vi "calculate_histogram.vi"(8 "error in (no error)":errorcluster, 9 "# bins [100]":i32=100, 10 "# std deviations for histogram width [1]":dbl=1.0, 11 "2D arr Intensity Graph":dbl[][](array[numeric])=array402x480[192960 elements]) -> (0 "error out":errorcluster, 1 "standard deviation":dbl format="%0.2f", 2 "mean":dbl format="%0.2f", 3 "Histogram Graph":T1(graph))   [LabVIEW 2019, in "graph_utilities.lvclass"]
uses:
  graph_utilities.lvclass
  <vilib>/Analysis/NI_AALPro.lvlib
  <vilib>/Analysis/NI_AALBase.lvlib
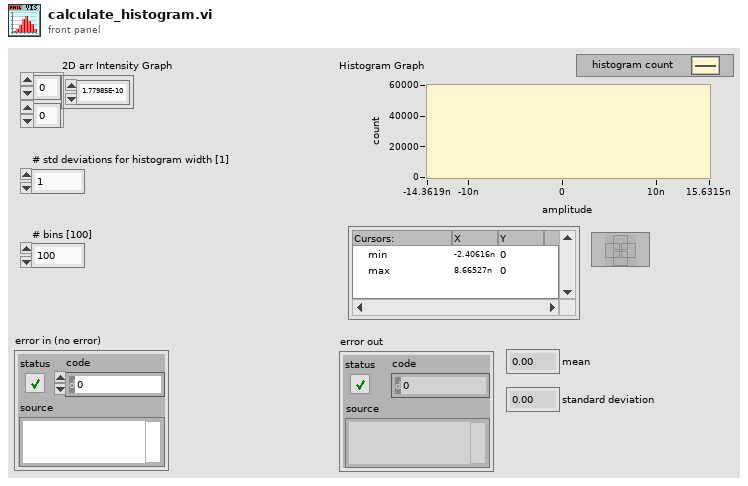
[diagram p1: front panel]
types:
  T1 = cluster{"X Values":dbl[], "Histogram: h(x)":i32[]}
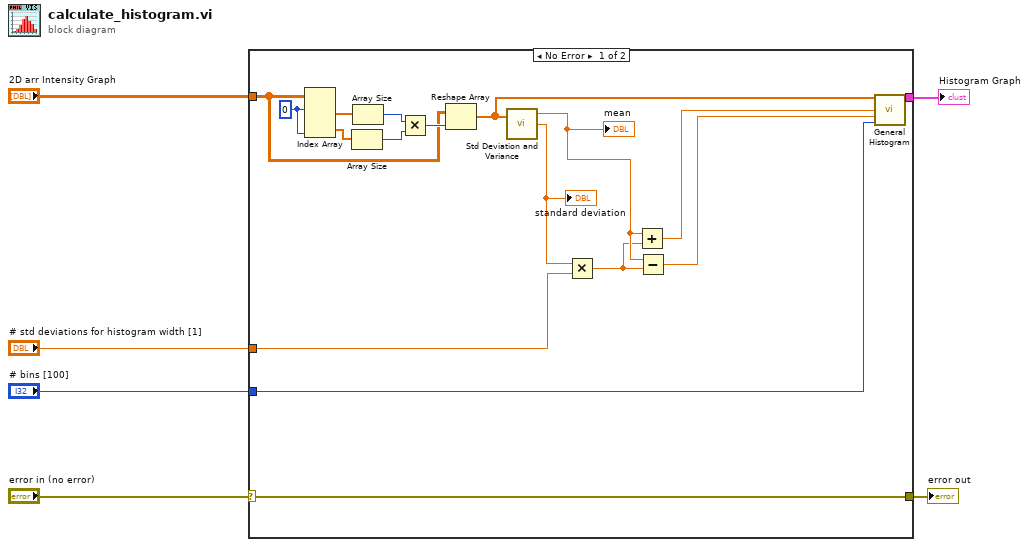
[diagram p0: block diagram]
diagram:
  n1 = case shown="No Error" "error in (no error)" {
    selector: "error in (no error)" -> [w7 w24]
    tunnel: "# std deviations for histogram width [1]" -> [w19 _]
    tunnel: "# bins [100]" -> [w13 _]
    tunnel: [w12 _] -> w4
    tunnel: "2D arr Intensity Graph" -> [w8 _]
    tunnel: [w7 w24] -> w1
    frame No Error {
      w16 = 0 ("index (row)")
      n2 = Index Array(array=w8, index (row) #1=w16, index (col) #2=w16) -> (element #1=w17:dbl[], element #2=w15:dbl[])  [unwired: 2 in]
      n3 = Array Size(array=w15) -> (size(s)=w9:i32)
      n4 = Array Size(array=w17) -> (size(s)=w10:i32)
      n5 = Multiply(x=w10, y=w9) -> (x*y=w14:i32)
      n6 = Reshape Array(w8, w14) -> (w11:dbl[])
      n7 = call <vilib>:"Std Deviation and Variance.vi"("X"=w11) -> ("mean"=w23:dbl, "standard deviation"=w20:dbl)  [unwired: 1 in, 1 out]
      "mean" <- w23
      "standard deviation" <- w20
      n8 = Multiply(x=w20, y=w19) -> (x*y=w18:dbl)
      n9 = Add(x=w23, y=w18) -> (x+y=w22:dbl)
      n10 = Subtract(x=w23, y=w18) -> (x-y=w21:dbl)
      n11 = call <vilib>:"General Histogram.vi"("X"=w11, "max"=w22, "min"=w21, "# bins"=w13) -> ("Histogram Graph"=w12:T1)  [unwired: 7 in, 4 out]
    }
    frame Error {
    }
  }
  "Histogram Graph" <- w4
  "error out" <- w1
